vi "Labels.vi"(7 "LabVIEW Web Service Request":refnum<class "Web Request.lvclass">) -> (2 "FuelLabels":T1(array[cluster]), 3 "TempLabels":string[][](array[string]))   [LabVIEW 2017]
uses:
  <vilib>/wsapi/Web Request.lvclass
panel:
  out "FuelLabels":string[][](array[string])
  # "Use the Web Service Request input terminal to call the VIs on the Web Services palette. Do not remove it from the connector pane unless you don't need access to the palette."
  # "Each additional control wired to the connector pane will be available as an input in the URL. To include an indicator in terminal-mode output (the default setting), it must also be wired to the connector pane."
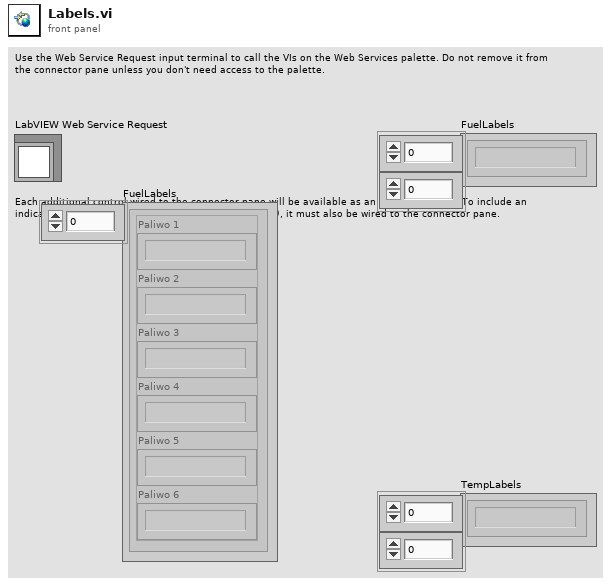
[diagram p1: front panel]
types:
  T1 = cluster{"Paliwo 1":string, "Paliwo 2":string, "Paliwo 3":string, "Paliwo 4":string, "Paliwo 5":string, "Paliwo 6":string}[]
  T2 = cluster{"Termometr 1":string, "Termometr 2":string, "Termometr 3":string, "Termometr 4":string, "Termometr 5":string, "Termometr 6":string, "Termometr 7":string, "Termometr 8":string, "Termometr 9":string, "Termometr 10":string}
  T3 = cluster{"Paliwo 1":string, "Paliwo 2":string, "Paliwo 3":string, "Paliwo 4":string, "Paliwo 5":string, "Paliwo 6":string}
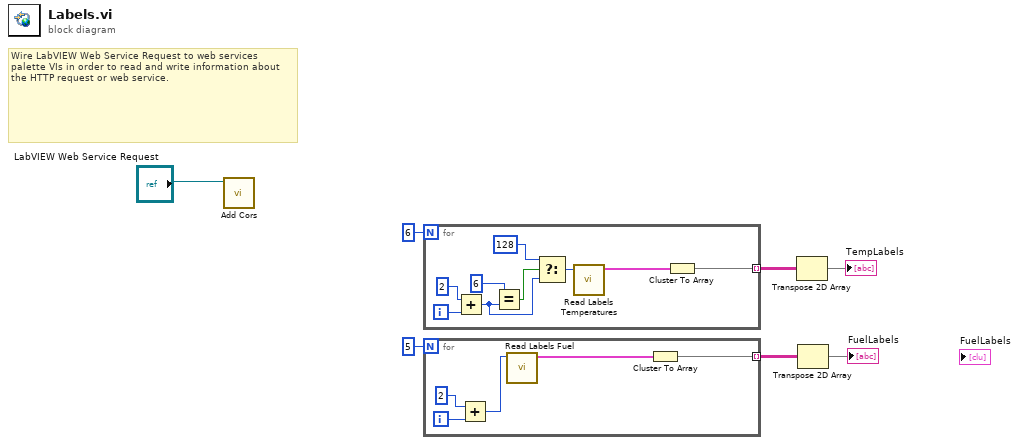
[diagram p0: block diagram]
diagram:
  # "Wire LabVIEW Web Service Request to web services palette VIs in order to read and write information about the HTTP request or web service."
  n1 = call "Add Cors.vi"("Web Request in"="LabVIEW Web Service Request") -> ()  [unwired: 10 in, 1 out]
  n2 = for {
    N: 6 -> [_]
    tunnel: [w8] -> w4 mode=indexing
    i -> [w16]
    n3 = Add(x=2, y=w16) -> (x+y=w11:i32)
    n4 = Equal?(x=6, y=w11) -> (x = y?=w12:bool)
    n5 = Select(t=128, s=w12, f=w11) -> (s? t:f=w14:i32)
    n6 = call "Read Labels Temperatures.vi"("Slave ID"=w14) -> ("Etykiety T1-10"=w9:T2)  [unwired: 10 in]
    n7 = Cluster To Array(cluster=w9) -> (array=w8:string[])
  }
  n8 = for {
    N: 5 -> [_]
    tunnel: [w17] -> w2 mode=indexing
    i -> [w21]
    n9 = Add(x=2, y=w21) -> (x+y=w19:i32)
    n10 = call "Read Labels Fuel.vi"("Slave ID"=w19) -> ("Etykiety P1-6"=w18:T3)  [unwired: 10 in]
    n11 = Cluster To Array(cluster=w18) -> (array=w17:string[])
  }
  n12 = Transpose 2D Array(2D array=w4) -> (transposed array=→"TempLabels":string[][])
  n13 = Transpose 2D Array(2D array=w2) -> (transposed array=→"FuelLabels":string[][])
